vi "Run.vi"(8 "error in (no error)":errorcluster, 9 "Penalty":dbl, 10 "Maze (0: Empty, -1: Enemy. >0: Teammate":i32[][](array[numeric])=[[16, 0, 18], [0, 14, 0], [0, 0, 0]], 11 "Borg In":refnum<class "Borg.lvclass">) -> (0 "error out":errorcluster, 1 "Direction":T1, 2 "Action":T2, 3 "Borg Out":refnum<class "Borg.lvclass">, 4 "Replicated":refnum<class "Square.lvclass">)   [LabVIEW 2015, in "Borg.lvclass"]
uses:
  Borg.lvclass
  Type Defs/Action Enum.ctl
  Type Defs/Direction Enum.ctl
  Square/Square.lvclass
  Borg.lvclass/Borg.ctl
  Type Defs/SB Type Defs.lvlib
  Common/Common.lvlib
panel:
  in  "Status":string
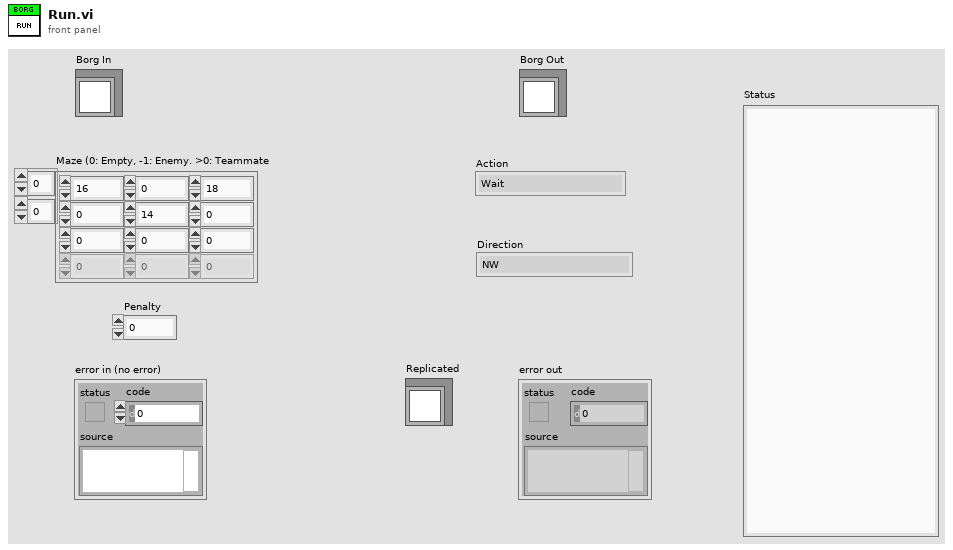
[diagram p1: front panel]
types:
  T1 = typedef "SB Type Defs.lvlib/Direction Enum.ctl" = enum16{"NW", "N", "NE", "E", "SE", "S", "SW", "W"}
  T2 = typedef "SB Type Defs.lvlib/Action Enum.ctl" = enum16{"Wait", "Move", "Attack", "Replicate"}
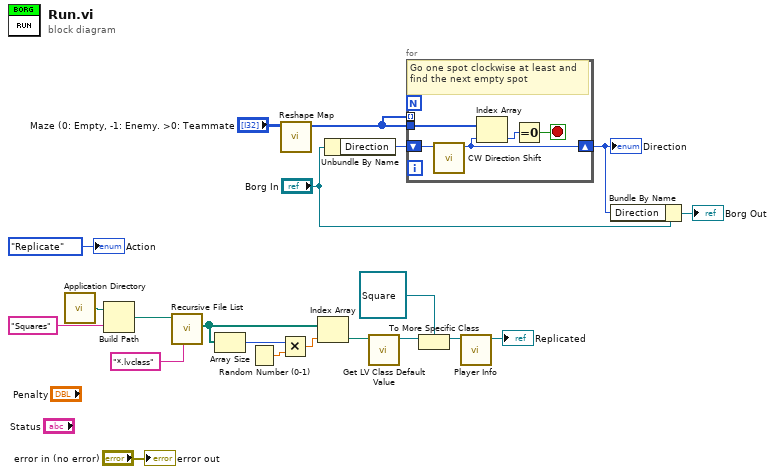
[diagram p0: block diagram]
diagram:
  n1 = call <vilib>:"Application Directory.vi"() -> ("Application Directory"=w15:path)
  n2 = Build Path(base path=w15, name or relative path="Squares") -> (appended path=w17:path)
  n3 = call <vilib>:"Recursive File List.vi"("pattern"="*.lvclass", "Folder Path"=w17) -> ("All Files in Dir"=w10:path[])  [unwired: 5 in, 4 out]
  n4 = Array Size(array=w10) -> (size(s)=w12:i32)
  n5 = Random Number (0-1)() -> (number: 0 to 1=w13:dbl)
  n6 = Multiply(x=w12, y=w13) -> (x*y=w8:dbl)
  n7 = call "Reshape Map.vi"("Maze (0: Empty, -1: Enemy. >0: Teammate"="Maze (0: Empty, -1: Enemy. >0: Teammate") -> ("Map"=w1:i32[])  [unwired: 9 in, 1 out]
  n8 = Index Array(array=w10, index=w8) -> (element=w9:path)
  n9 = Unbundle By Name("Borg In") -> ("Direction"=w3:T1)
  n10 = call <vilib>:"Get LV Class Default Value.vi"("class path"=w9) -> ("object"=w18:refnum<class>)  [unwired: 9 in, 1 out]
  n11 = for {
    shift-right: [w25] -> w2
    shift-left: w3 -> [w26]
    tunnel: w1 -> [w24]
    tunnel: w1 -> [_] mode=indexing
    stop <- w22 stop-if-true
    # "Go one spot clockwise at least and find the next empty spot"
    n12 = call "CW Direction Shift.vi"("Direction"=w26) -> ("Numeric"=w25:i32)  [unwired: 10 in]
    n13 = Index Array(array=w24, index=w25) -> (element=w23:i32)
    n14 = Equal To 0?(x=w23) -> (x = 0?=w22:bool)
  }
  "Direction" <- w2
  n15 = To More Specific Class(target class=refnum<class "Square.lvclass"> refnum ("Runner.lvclass"), reference=w18) -> (specific class reference=w20:refnum<class "Square.lvclass">)  [unwired: 1 in, 1 out]
  n16 = call-dynamic "Player Info.vi"("Square in"=w20) -> ("Square out"=→"Replicated":refnum<class "Square.lvclass">)  [unwired: 8 in, 2 out]
  n17 = Bundle By Name(cluster="Borg In", "Direction"=w2) -> (→"Borg Out":refnum<class "Borg.lvclass">)
  "error out" <- "error in (no error)"
  "Action" <- Action_Enum."Replicate" ("Action")
